vi "自动保存TXT.vi"(0 "MCListbox引用句柄":refnum<vi>) -> ()   [LabVIEW 2014]
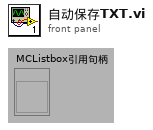
[diagram p1: front panel]
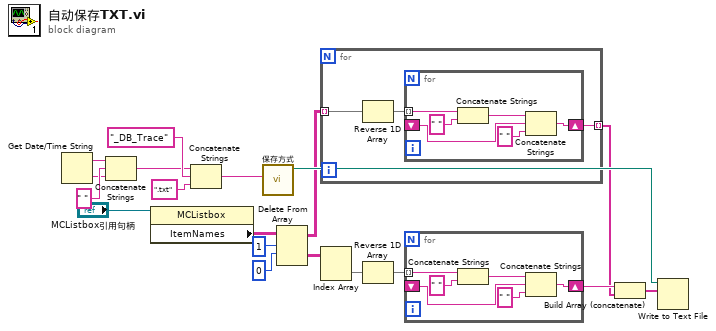
[diagram p0: block diagram]
diagram:
  n1 = Get Date/Time String() -> (date string=w12:string, time string=w13:string)  [unwired: 3 in]
  n2 = Concatenate Strings(w12, " " ("字符串"), w13) -> (w14:string)
  n3 = property on="属性节点" class="MCListbox"(reference="MCListbox引用句柄") -> ("ItemNames"=w2:string[][])  [unwired: 1 in, 2 out]
  n4 = Concatenate Strings(w14, "_DB_Trace" ("字符串"), ".txt" ("名称或相对路径")) -> (w17:string)
  n5 = call "保存方式.vi"("名称或相对路径"=w17) -> ("添加的路径"=w19:path)  [unwired: 10 in]
  n6 = Delete From Array(array=w2, length=1 ("长度"), index (row)=0 ("索引 (行)")) -> (deleted portion=w9:string[][], array with subset deleted=w5:string[][])  [unwired: 1 in]
  n7 = for {
    tunnel: w5 -> [w21] mode=indexing
    tunnel: [w20] -> w4 mode=indexing
    n8 = Reverse 1D Array(array=w21) -> (reversed array=w22:string[])
    n9 = for {
      tunnel: w22 -> [w27] mode=indexing
      shift-right: [w24] -> w20
      shift-left: _ -> [w26]
      n10 = Concatenate Strings(w27, " " ("字符串")) -> (w25:string)
      n11 = Concatenate Strings(w25, w26, " " ("字符串")) -> (w24:string)
    }
  }
  n12 = Index Array(array=w9) -> (element=w7:string[])  [unwired: 2 in]
  n13 = Reverse 1D Array(array=w7) -> (reversed array=w6:string[])
  n14 = for {
    tunnel: w6 -> [w33] mode=indexing
    shift-right: [w30] -> w8
    shift-left: _ -> [w32]
    n15 = Concatenate Strings(w33, " " ("字符串")) -> (w31:string)
    n16 = Concatenate Strings(w31, w32, " " ("字符串")) -> (w30:string)
  }
  n17 = Build Array (concatenate)(w8, w4) -> (w3:string[])
  n18 = Write to Text File(file (use dialog)=w19, text=w3) -> ()  [unwired: 2 in, 3 out]
